vi "test Receive Message.vi"(8 "error in (no error)":errorcluster, 11 "TestCase in":refnum<class "Test TCP Stream Transmission.lvclass">) -> (0 "error out":errorcluster, 3 "TestCase out":refnum<class "Test TCP Stream Transmission.lvclass">)   [LabVIEW 2020, in "Test TCP Stream Transmission.lvclass"]
uses:
  Test TCP Stream Transmission.lvclass
  <vilib>/addons/_JKI Toolkits/VI Tester/TestCase.llb/TestCase.lvclass
  <vilib>/ActorFramework/LastAck/Last Ack.lvclass
  Source/Protocols/TCP Strategy/TCP Stream Initiator/TCP Stream Initiator.lvclass
  Source/Abstract Classes/Cipher/Cipher.lvclass
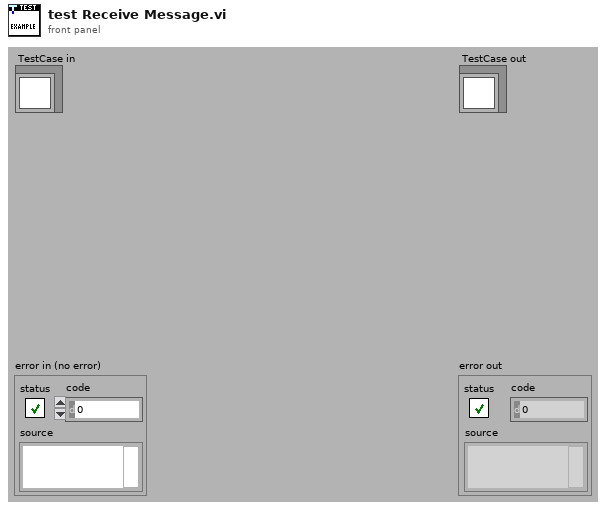
[diagram p1: front panel]
types:
  T1 = cluster{"Last Ack":refnum<class "Last Ack.lvclass">, "priority":i32}
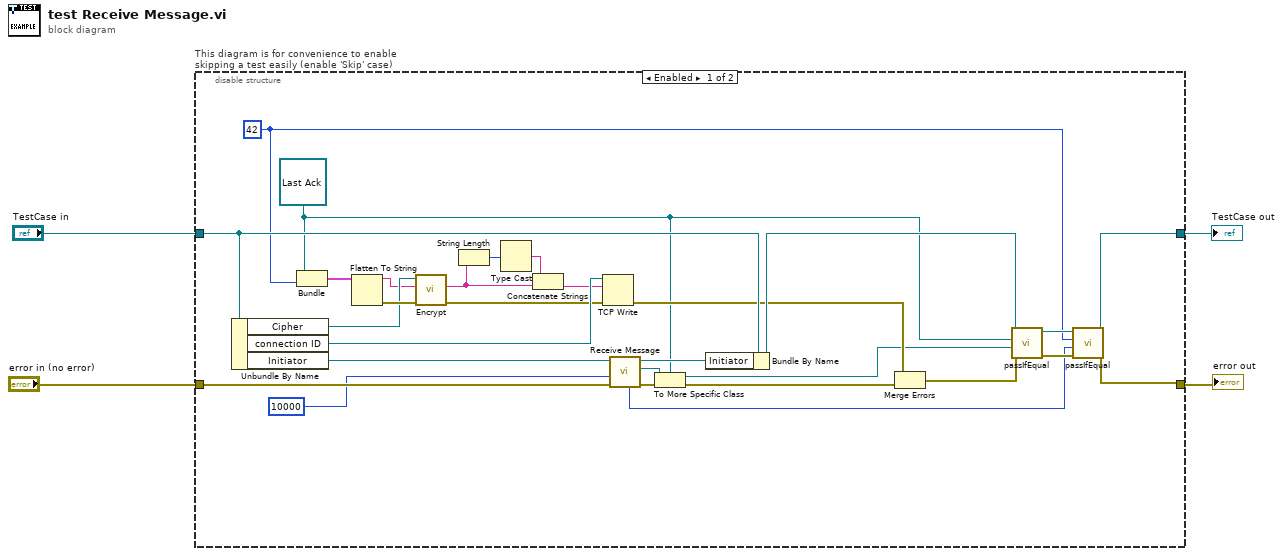
[diagram p0: block diagram]
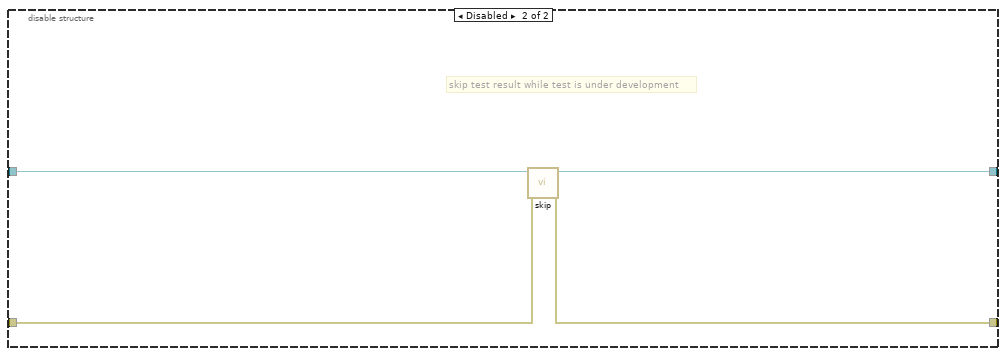
[diagram p2: hidden frame]
diagram:
  n1 = disable-structure "This diagram is for convenience to enable skipping a test easily (enable 'Skip' case)" shown="Enabled" {
    disable-tunnel: "TestCase in" -> [w30 w37]
    disable-tunnel: [w13 w35] -> w1
    disable-tunnel: [w15 w36] -> w3
    disable-tunnel: "error in (no error)" -> [w33 w34]
    frame Enabled {
      w12 = 42 ("priority")
      w18 = refnum<class "Last Ack.lvclass"> refnum ("Last Ack")
      n2 = Unbundle By Name(w30) -> ("Cipher"=w8:refnum<class "Cipher.lvclass">, "connection ID"=w23:refnum<k5>, "Initiator"=w32:refnum<class "TCP Stream Initiator.lvclass">)
      n3 = Bundle("Last Ack"=w18, "priority"=w12) -> (w17:T1)  [unwired: 1 in]
      n4 = Flatten To String(anything=w17) -> (data string=w7:string, error out=w10:errorcluster)  [unwired: 3 in, 1 out]
      n5 = call-dynamic "Encrypt.vi"("error in (no error)"=w10, "Plaintext"=w7, "Cipher in"=w8) -> ("error out"=w9:errorcluster, "Cyphertext"=w6:string)  [unwired: 6 in, 1 out]
      n6 = String Length(string=w6) -> (length=w26:i32)
      n7 = Type Cast(x=w26) -> (*(type *) &x=w27:string)  [unwired: 1 in]
      n8 = Concatenate Strings(w27, w6) -> (w5:string)
      n9 = TCP Write(connection ID=w23, data in=w5, error in (no error)=w9) -> (error out=w24:errorcluster)  [unwired: 1 in, 2 out]
      n10 = call-dynamic "Receive Message.vi"("error in (no error)"=w33, "timeout ms (-1)"=10000, "TCP Stream in"=w32) -> ("error out"=w22:errorcluster, "Message"=w20:refnum<class "Message.lvclass">, "TCP Stream out"=w31:refnum<class "TCP Stream Initiator.lvclass">, "priority"=w11:i32)  [unwired: 4 in, 1 out]
      n11 = To More Specific Class(target class=w18, reference=w20, error in=w22) -> (specific class reference=w19:refnum<class "Last Ack.lvclass">, error out=w21:errorcluster)
      n12 = Bundle By Name(cluster=w30, "Initiator"=w31) -> (w29:refnum<class "Test TCP Stream Transmission.lvclass">)
      n13 = Merge Errors(w24, w21) -> (w25:errorcluster)
      n14 = call-dynamic "passIfEqual.vi"("error in (no error)"=w25, "y"=w19, "x"=w18, "TestCase in"=w29) -> ("error out"=w16:errorcluster, "TestCase out"=w14:refnum<class "Test TCP Stream Transmission.lvclass">)  [unwired: 6 in]
      n15 = call-dynamic "passIfEqual.vi"("error in (no error)"=w16, "y"=w11, "x"=w12, "TestCase in"=w14) -> ("error out"=w15:errorcluster, "TestCase out"=w13:refnum<class "Test TCP Stream Transmission.lvclass">)  [unwired: 6 in]
    }
    frame Disabled {
      # "skip test result while test is under development"
      n16 = call <vilib>:"skip.vi"("error in (no error)"=w34, "TestCase in"=w37) -> ("error out"=w36:errorcluster, "TestCase out"=w35:refnum<class "Test TCP Stream Transmission.lvclass">)  [unwired: 8 in]
    }
  }
  "error out" <- w3
  "TestCase out" <- w1
